vi "GDSFIle_ConvertLLBs.vi"(8 "error in (no error)":errorcluster, 11 "ClassPath Or LLB Path":path) -> (0 "error out":errorcluster, 3 "ClassPath Or LLB Path Out":path)   [LabVIEW 2020]
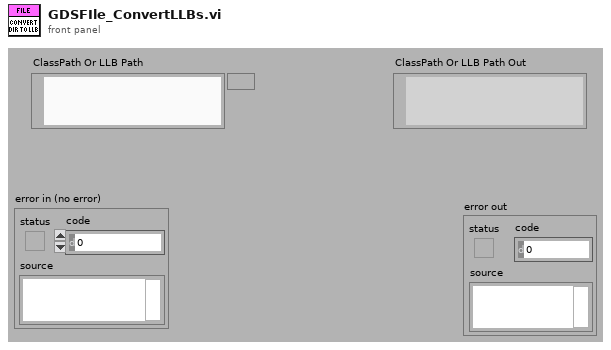
[diagram p1: front panel]
types:
  T1 = cluster{"Temporary LLB":path, "Final LLB":path, "Source Directory":path}
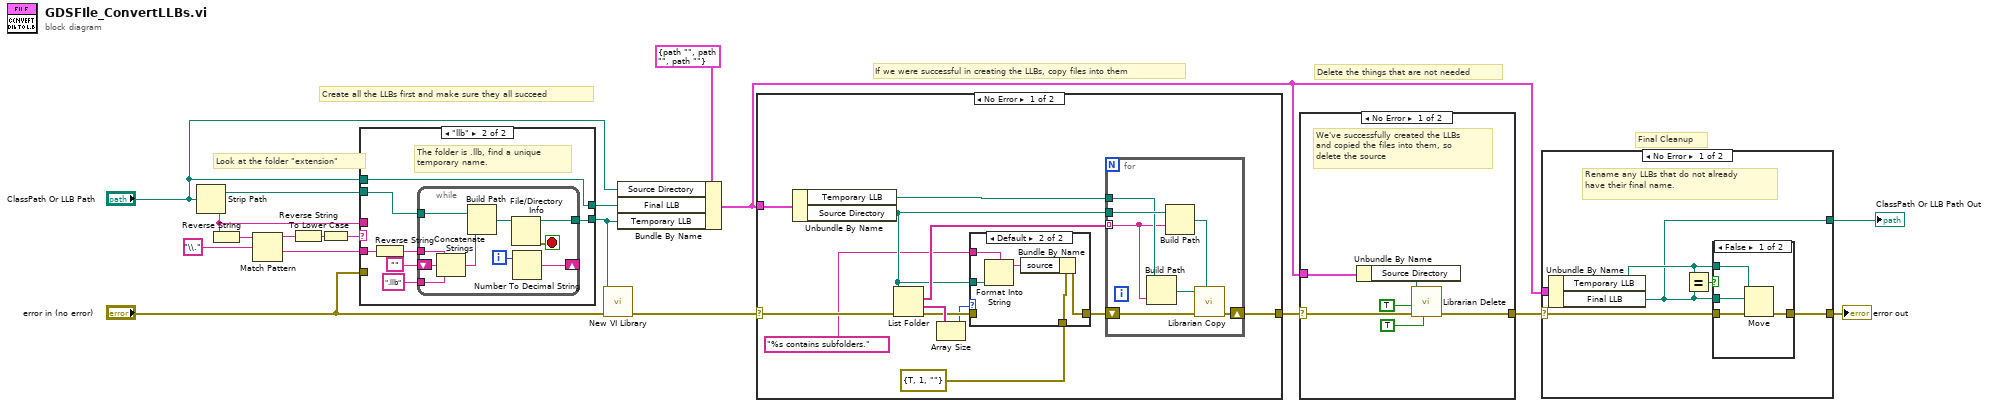
[diagram p0: block diagram]
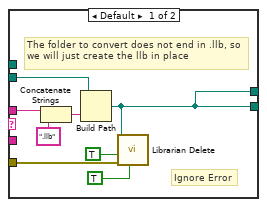
[diagram p2: hidden frame]
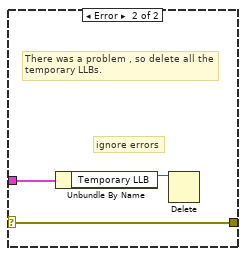
[diagram p5: hidden frame]
diagram:
  # "Look at the folder \"extension\""
  # "Final Cleanup"
  # "Delete the things that are not needed"
  # "If we were successful in creating the LLBs, copy files into them"
  # "Create all the LLBs first and make sure they all succeed"
  n1 = Strip Path(path="ClassPath Or LLB Path") -> (stripped path=w6:path, name=w7:string)
  n2 = Reverse String(1:w7) -> (0:w11:string)
  n3 = Match Pattern(string=w11, regular expression="\\.") -> (before substring=w4:string, after substring=w3:string)  [unwired: 1 in, 2 out]
  n4 = Reverse String(1:w4) -> (0:w9:string)
  n5 = To Lower Case(string=w9) -> (all lower case string=w8:string)
  n6 = case shown="\"llb\"" w8 {
    tunnel: w3 -> [_ w34]
    tunnel: w7 -> [w20 _]
    tunnel: w6 -> [w25 w31]
    tunnel: [w24 w28] -> w2
    tunnel: [w24 w29] -> w5
    tunnel: "ClassPath Or LLB Path" -> [_ w29]
    tunnel: "error in (no error)" -> [w22 _]
    frame Default {
      # "Ignore Error"
      # "The folder to convert does not end in .llb, so we will just create the llb in place"
      n7 = Concatenate Strings(w20, ".llb" ("string")) -> (w26:string)
      n8 = Build Path(base path=w25, name or relative path=w26) -> (appended path=w24:path)
      n9 = call <vilib>:"Librarian Delete.vi"("keep deleting on error? (F)"=TRUE, "error in (no error)"=w22, "recursive? (F)"=TRUE, "path"=w24) -> ()  [unwired: 7 in, 1 out]
    }
    frame "llb" {
      # "The folder is .llb, find a unique temporary name."
      n10 = Reverse String(1:w34) -> (0:w33:string)
      n11 = while {
        tunnel: w33 -> [w43]
        shift-right: [w39] -> _
        shift-left: "" -> [w44]
        tunnel: w31 -> [w41]
        tunnel: [w36] -> w28
        tunnel: ".llb" ("string") -> [w35]
        i -> [w40]
        stop <- w37 stop-if-true
        n12 = Concatenate Strings(w43, w44, w35) -> (w42:string)
        n13 = Build Path(base path=w41, name or relative path=w42) -> (appended path=w38:path)
        n14 = File/Directory Info(path=w38) -> (path out=w36:path, error out=w37:errorcluster)  [unwired: 1 in, 5 out]
        n15 = Number To Decimal String(number=w40) -> (decimal integer string=w39:string)  [unwired: 1 in]
      }
    }
  }
  n16 = call <vilib>:"New VI Library.vi"("error in (no error)"="error in (no error)", "VI library path in"=w2) -> ("error out"=w16:errorcluster)  [unwired: 8 in, 1 out]
  n17 = Bundle By Name(cluster=T1 {"Temporary LLB"=path "", "Final LLB"=path "", "Source Directory"=path ""}, "Source Directory"="ClassPath Or LLB Path", "Final LLB"=w5, "Temporary LLB"=w2) -> (w12:T1)
  n18 = case shown="No Error" w16 {
    selector: w16 -> [w56 w70]
    tunnel: w12 -> [w54 _]
    tunnel: [w55 w70] -> w15
    frame No Error {
      n19 = Unbundle By Name(w54) -> ("Temporary LLB"=w49:path, "Source Directory"=w47:path)
      n20 = List Folder(path=w47, error in=w56) -> (filenames=w50:string[], folder names=w52:string[], error out=w51:errorcluster)  [unwired: 2 in, 1 out]
      n21 = Array Size(array=w52) -> (size(s)=w46:i32)
      n22 = case shown="Default" w46 {
        tunnel: w47 -> [_ w69]
        tunnel: [w64 w66] -> w48
        tunnel: w51 -> [w64 _]
        tunnel: errorcluster {"status"=TRUE, "code"=1, "source"=""} ("error IO") -> [_ w67]
        tunnel: "%s contains subfolders." ("Contains Folders") -> [_ w65]
        frame 0 {
          # "Directory has no subdirs"
        }
        frame Default {
          n23 = Format Into String(format string=w65, w69) -> (resulting string=w68:string)  [unwired: 2 in, 1 out]
          n24 = Bundle By Name(cluster=w67, "source"=w68) -> (w66:errorcluster)
        }
      }
      n25 = for {
        tunnel: w50 -> [w60] mode=indexing
        tunnel: w47 -> [w63]
        tunnel: w49 -> [w61]
        shift-right: [w57] -> w55
        shift-left: w48 -> [w58]
        n26 = Build Path(base path=w61, name or relative path=w60) -> (appended path=w59:path)
        n27 = Build Path(base path=w63, name or relative path=w60) -> (appended path=w62:path)
        n28 = call <vilib>:"Librarian Copy.vi"("source"=w62, "error in (no error)"=w58, "destination"=w59) -> ("error out"=w57:errorcluster)  [unwired: 7 in, 1 out]
      }
    }
    frame Error {
    }
  }
  n29 = case shown="No Error" w15 {
    selector: w15 -> [w76 w79]
    tunnel: w12 -> [w75 w78]
    tunnel: [w74 w79] -> w14
    frame No Error {
      # "We've successfully created the LLBs and copied the files into them, so delete the source"
      n30 = Unbundle By Name(w75) -> ("Source Directory"=w73:path)
      n31 = call <vilib>:"Librarian Delete.vi"("keep deleting on error? (F)"=TRUE, "error in (no error)"=w76, "recursive? (F)"=TRUE, "path"=w73) -> ("error out"=w74:errorcluster)  [unwired: 7 in]
    }
    frame Error {
      # "ignore errors"
      # "There was a problem , so delete all the temporary LLBs."
      n32 = Unbundle By Name(w78) -> ("Temporary LLB"=w77:path)
      n33 = Delete(path (use dialog)=w77) -> ()  [unwired: 4 in, 3 out]
    }
  }
  n34 = case shown="No Error" w14 {
    selector: w14 -> [w84 w91]
    tunnel: w12 -> [w85 _]
    tunnel: [w83 w91] -> w13
    tunnel: [w80 _] -> w1
    frame No Error {
      # "Rename any LLBs that do not already have their final name."
      n35 = Unbundle By Name(w85) -> ("Temporary LLB"=w81:path, "Final LLB"=w80:path)
      n36 = Equal?(x=w81, y=w80) -> (x = y?=w82:bool)
      n37 = case shown="False" w82 {
        tunnel: w81 -> [w89 _]
        tunnel: w80 -> [w88 _]
        tunnel: w84 -> [w87 w90]
        tunnel: [w86 w90] -> w83
        frame False {
          n38 = Move(source path=w89, error in=w87, 10:w88) -> (error out=w86:errorcluster)  [unwired: 2 in, 2 out]
        }
        frame True {
        }
      }
    }
    frame Error {
    }
  }
  "error out" <- w13
  "ClassPath Or LLB Path Out" <- w1
